vi "ToGraphChart.vi"(8 "error in":errorcluster, 11 "Generic in":refnum<class "Generic.lvclass">) -> (0 "error out":errorcluster, 3 "GraphChart out":refnum<class "GraphChart.lvclass">)   [LabVIEW 2014, in "GraphChart.lvclass"]
uses:
  GraphChart.lvclass
  Generic/Generic.lvclass
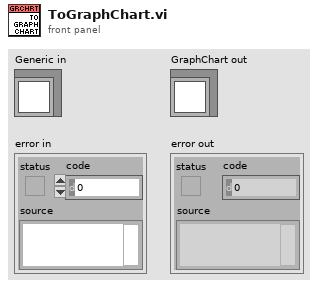
[diagram p1: front panel]
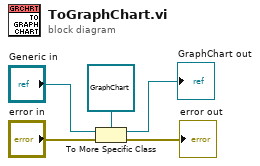
[diagram p0: block diagram]
diagram:
  n1 = To More Specific Class(target class=refnum<class "GraphChart.lvclass"> refnum ("RotaryColorScale in 2"), reference="Generic in", error in="error in") -> (specific class reference=→"GraphChart out":refnum<class "GraphChart.lvclass">, error out=→"error out":errorcluster)
